vi "SMO.Example.SetState.vi"(8 "error in (no error)":errorcluster, 10 "Pump State":bool, 11 "SMO.Example":refnum<class "SMO.Example.lvclass">) -> (0 "error out":errorcluster, 3 "SMO.Example out":refnum<class "SMO.Example.lvclass">)   [LabVIEW 2013, in "SMO.Example.lvclass"]
doc: "---------------------------------------------------------------\nJKI State Machine Objects™\nhttp://jki.net/state-machine-objects/\nCopyright (C) 2005-2015, JKI <info@jki.net>\nALL RIGHTS RESERVED"
uses:
  SMO.Example.lvclass
panel:
  # "For instructions on how to use the JKI State Machine Objects, examples and video tutorials, visit:\nhttp://jki.net/state-machine-objects/\n\nJKI State Machine Objects™\nhttp://jki.net/state-machine-objects/\nCopyright (C) 2005-2015, JKI <info@jki.net>\nALL RIGHTS RESERVED"
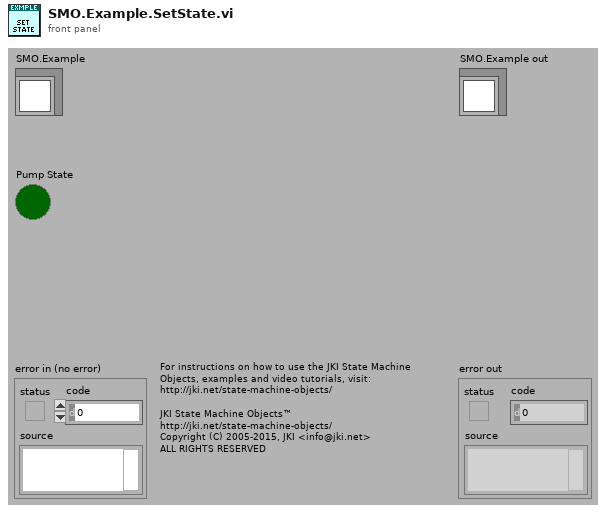
[diagram p1: front panel]
types:
  T1 = typedef "SMO.Example.lvclass/PublicEvents--Cluster.ctl" = cluster{"Data Changed":refnum<user-event>, "State Changed":refnum<user-event>}
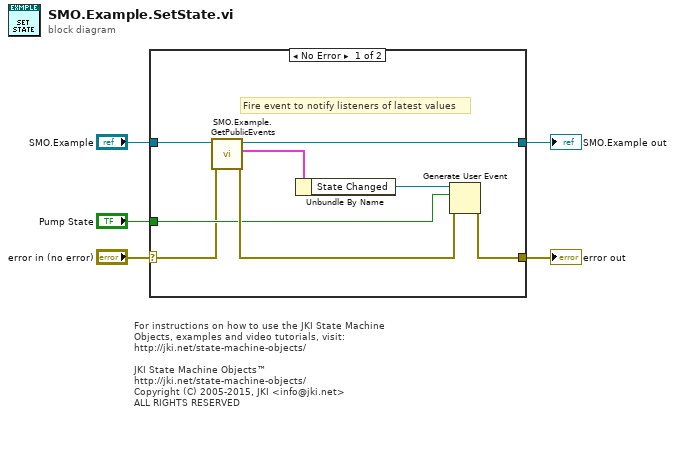
[diagram p0: block diagram]
diagram:
  # "For instructions on how to use the JKI State Machine Objects, examples and video tutorials, visit:\nhttp://jki.net/state-machine-objects/\n\nJKI State Machine Objects™\nhttp://jki.net/state-machine-objects/\nCopyright (C) 2005-2015, JKI <info@jki.net>\nALL RIGHTS RESERVED"
  n1 = case shown="No Error" "error in (no error)" {
    selector: "error in (no error)" -> [w6 w14]
    tunnel: "SMO.Example" -> [w8 w15]
    tunnel: [w9 w14] -> w4
    tunnel: [w13 w15] -> w3
    tunnel: "Pump State" -> [w7 _]
    frame No Error {
      # "Fire event to notify listeners of latest values"
      n2 = call "SMO.Example.GetPublicEvents.vi"("error in (no error)"=w6, "SMO.Example"=w8) -> ("error out"=w10:errorcluster, "SMO.Example Public Events"=w12:T1, "SMO.Example out"=w13:refnum<class "SMO.Example.lvclass">)  [unwired: 7 in]
      n3 = Unbundle By Name(w12) -> ("State Changed"=w11:refnum<user-event>)
      n4 = Generate User Event(user event=w11, event data cluster=w7, error in=w10) -> (error out=w9:errorcluster)  [unwired: 1 in, 1 out]
    }
    frame Error {
    }
  }
  "error out" <- w4
  "SMO.Example out" <- w3
